vi "Get Marker Value.vi"(4 "error in (no error)":errorcluster, 7 "VISA resource name":refnum<visa-resource-name>) -> (0 "error out":errorcluster, 1 "read buffer":string, 2 "Marker Value":dbl, 3 "VISA resource name out":refnum<visa-resource-name>)   [LabVIEW 2015]
doc: "Requests the active marker values in 3 numbers from the HP8753C Network Analyser. The first two numbers are the marker values, and the last is the stimulus value (these can all be seen on the read buffer output). It then extracts the first value and outputs this as Marker Value"
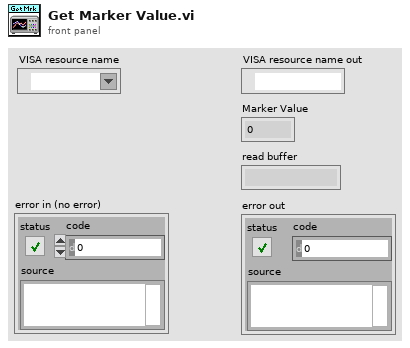
[diagram p1: front panel]
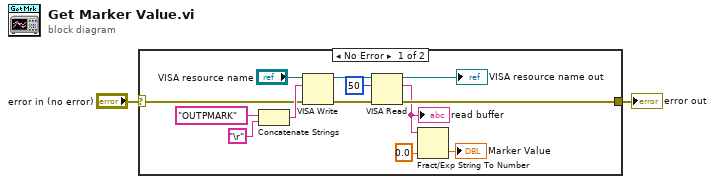
[diagram p0: block diagram]
diagram:
  n1 = case shown="No Error" "error in (no error)" {
    selector: "error in (no error)" -> [w3 w16]
    tunnel: [w7 w16] -> w2
    frame No Error {
      n2 = Concatenate Strings("OUTPMARK", "\r") -> (w10:string)
      n3 = VISA Write(VISA resource name="VISA resource name", write buffer=w10, error in (no error)=w3) -> (VISA resource name out=w14:refnum<visa-resource-name>, error out=w15:errorcluster)  [unwired: 1 out]
      n4 = VISA Read(VISA resource name=w14, byte count=u32 50, error in (no error)=w15) -> (VISA resource name out=→"VISA resource name out":refnum<visa-resource-name>, read buffer=w4:string, error out=w7:errorcluster)  [unwired: 1 out]
      "read buffer" <- w4
      n5 = Fract/Exp String To Number(string=w4, default (0 dbl)=0.0) -> (number=→"Marker Value":dbl)  [unwired: 2 in, 1 out]
    }
    frame Error {
    }
  }
  "error out" <- w2
